vi "St temp2.vi"(11 "Station Name":string) -> ()   [LabVIEW 2019]
uses:
  Ctrl/Conveyor Action.ctl
  <vilib>/Utility/miscctls.llb/LVPointTypeDef.ctl
  Ctrl/Auto Inspection Data Name.ctl
  Ctrl/Auto Inspection Station Name2.ctl
  LLB/Message/Ctrl/MsgDataInput.ctl
  LLB/Message/Ctrl/MsgPageSelect.ctl
  LLB/Message/Ctrl/LogType.ctl
  9b7d8055-4de2-48cf-bbcb-f861e34e7884.vi
  2931b48d-cced-43b2-9067-584d882f955d.vi
  <vilib>/JDP Science/JSONtext/Variant to JSON Text.vi
  <vilib>/JDP Science/JSONtext/JSON text to Variant.vi
  LLB/Commonly VI.lvlib
  ab69a899-d2ec-4c26-af5e-ed1cd18d461c.vi
  Function/Axis/Axis_Class/SubVI/Axis Motion/Axis_Go Home.vi
  LLB/Message/MsgShowAndLog.lvlib
panel:
  in  "Table Control":string[][](table)
  out "Station Name 3":string
  in  "Enum 2":T1
  in  "Cluster":cluster{"Enum 2":T1, "Station Name 3":string}
  in  "CurrentAction":string
  in  "Status":string
  in  "Errset":bool
  out "Message":string
  out "Ring":u16(ring)
  in  "Btn_AutoRun":bool
  in  "Boolean":bool=TRUE
  in  "Btn_Home":bool
  in  "AI":T2
  in  "Tab Control":enum32{"Page 1", "Page 2"}(tab)
  in  "Enum 28":T1
  out "Station Name 29":string
  in  "Enum 27":T1
  out "Station Name 28":string
  in  "Enum 26":T1
  out "Station Name 27":string
  in  "Enum 25":T1
  out "Station Name 26":string
  in  "Enum 24":T1
  out "Station Name 25":string
  in  "Enum 23":T1
  out "Station Name 24":string
  in  "Enum 22":T1
  out "Station Name 23":string
  in  "Enum 21":T1
  out "Station Name 22":string
  in  "Enum 20":T1
  out "Station Name 21":string
  out "Station Name 19":string
  in  "Enum 18":T1
  out "Station Name 18":string
  in  "Enum 17":T1
  out "Station Name 17":string
  in  "Enum 16":T1
  out "Station Name 16":string
  in  "Enum 15":T1
  out "Station Name 15":string
  in  "Enum 14":T1
  out "Station Name 14":string
  in  "Enum 13":T1
  out "Station Name 13":string
  in  "Enum 12":T1
  out "Station Name 12":string
  in  "Enum 11":T1
  out "Station Name 11":string
  in  "Enum 10":T1
  out "Station Name 10":string
  in  "Enum 9":T1
  out "Station Name 9":string
  in  "Enum 8":T1
  out "Station Name 8":string
  in  "Enum 7":T1
  out "Station Name 7":string
  in  "Enum 6":T1
  out "Station Name 6":string
  in  "Enum 5":T1
  out "Station Name 5":string
  in  "Enum 4":T1
  out "Station Name 4":string
  in  "Enum 3":T1
  in  "Enum 19":T1
  out "Station Name 20":string
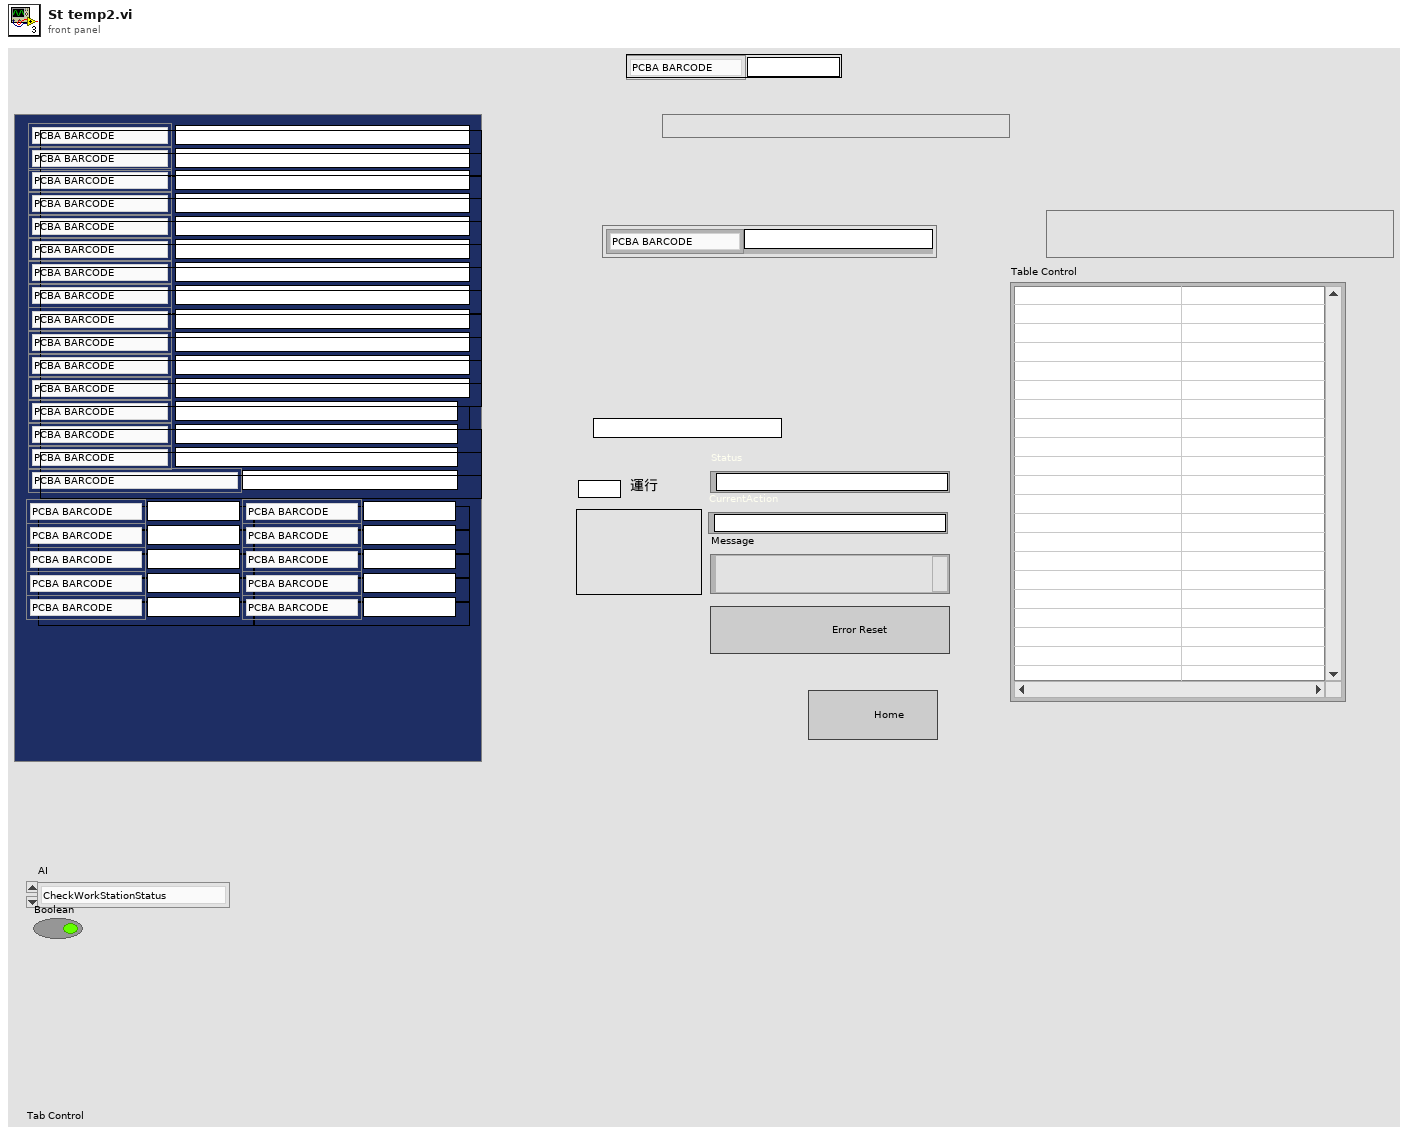
[diagram p1: front panel]
types:
  T1 = typedef "名稱資訊.ctl" = enum16{"PCBA BARCODE", "硬體(Tool初始化)", "company(Tool初始化)", "耗電流 uA(電流表)", "電池負載電壓", "晶片ID(Tool FORMAT)", "雷雕ID", "Format Status", "Programe Status", "MAC(藍芽接收器)", "ID(藍芽接收器)", "KPA(藍芽接收器)", "溫度(藍芽接收器)", "BattVol(藍芽接收器)", "RSSI(藍芽接收器)"}
  T2 = typedef "Conveyor Action.ctl" = enum16{"CheckWorkStationStatus", "Request Item In", "Check Product Ready In", "Wait Item In", "Check SlowSignal And Slow", "Check Arrive", "Rise Tray", "FixTray", "Imform Robot", "Wait Robot Imform", "DropTray Imform Out", "Wait Request ", "Flow Out"}
  T3 = enum8{"Enabled", "Disabled", "Disabled and Grayed Out"}
  T4 = typedef "LVPointTypeDef.ctl" = cluster{"Horizontal":i16, "Vertical":i16}
  T5 = typedef "MsgDataInput.ctl" = cluster{"MsgPageSelect":T6, "LogType":T7, "Msg":string, "Time":string}
  T6 = typedef "MsgShowAndLog.lvlib/MsgPageSelect.ctl" = enum16{"System", "Comm", "IO", "Action", "Alarm"}
  T7 = typedef "MsgShowAndLog.lvlib/LogType.ctl" = enum16{"Auto", "Manual", "Handshake", "Error"}
  T8 = typedef "Auto Inspection Station Name2.ctl" = enum16{"S1Barcode", "S2Measure", "S3Measure", "S4Measure", "S5Measure", "S11_LaserCheck"}
  T9 = typedef "Auto Inspection Data Name.ctl" = enum16{"LocalRun", "ItemSN(TimeCode)", "CurrentAction", "Error", "Data", "OKNG", "電壓值", "電壓值判斷", "電流值", "電流值判斷", "Laser Data", "Laser OK", "Laser NG", "StationNO"}
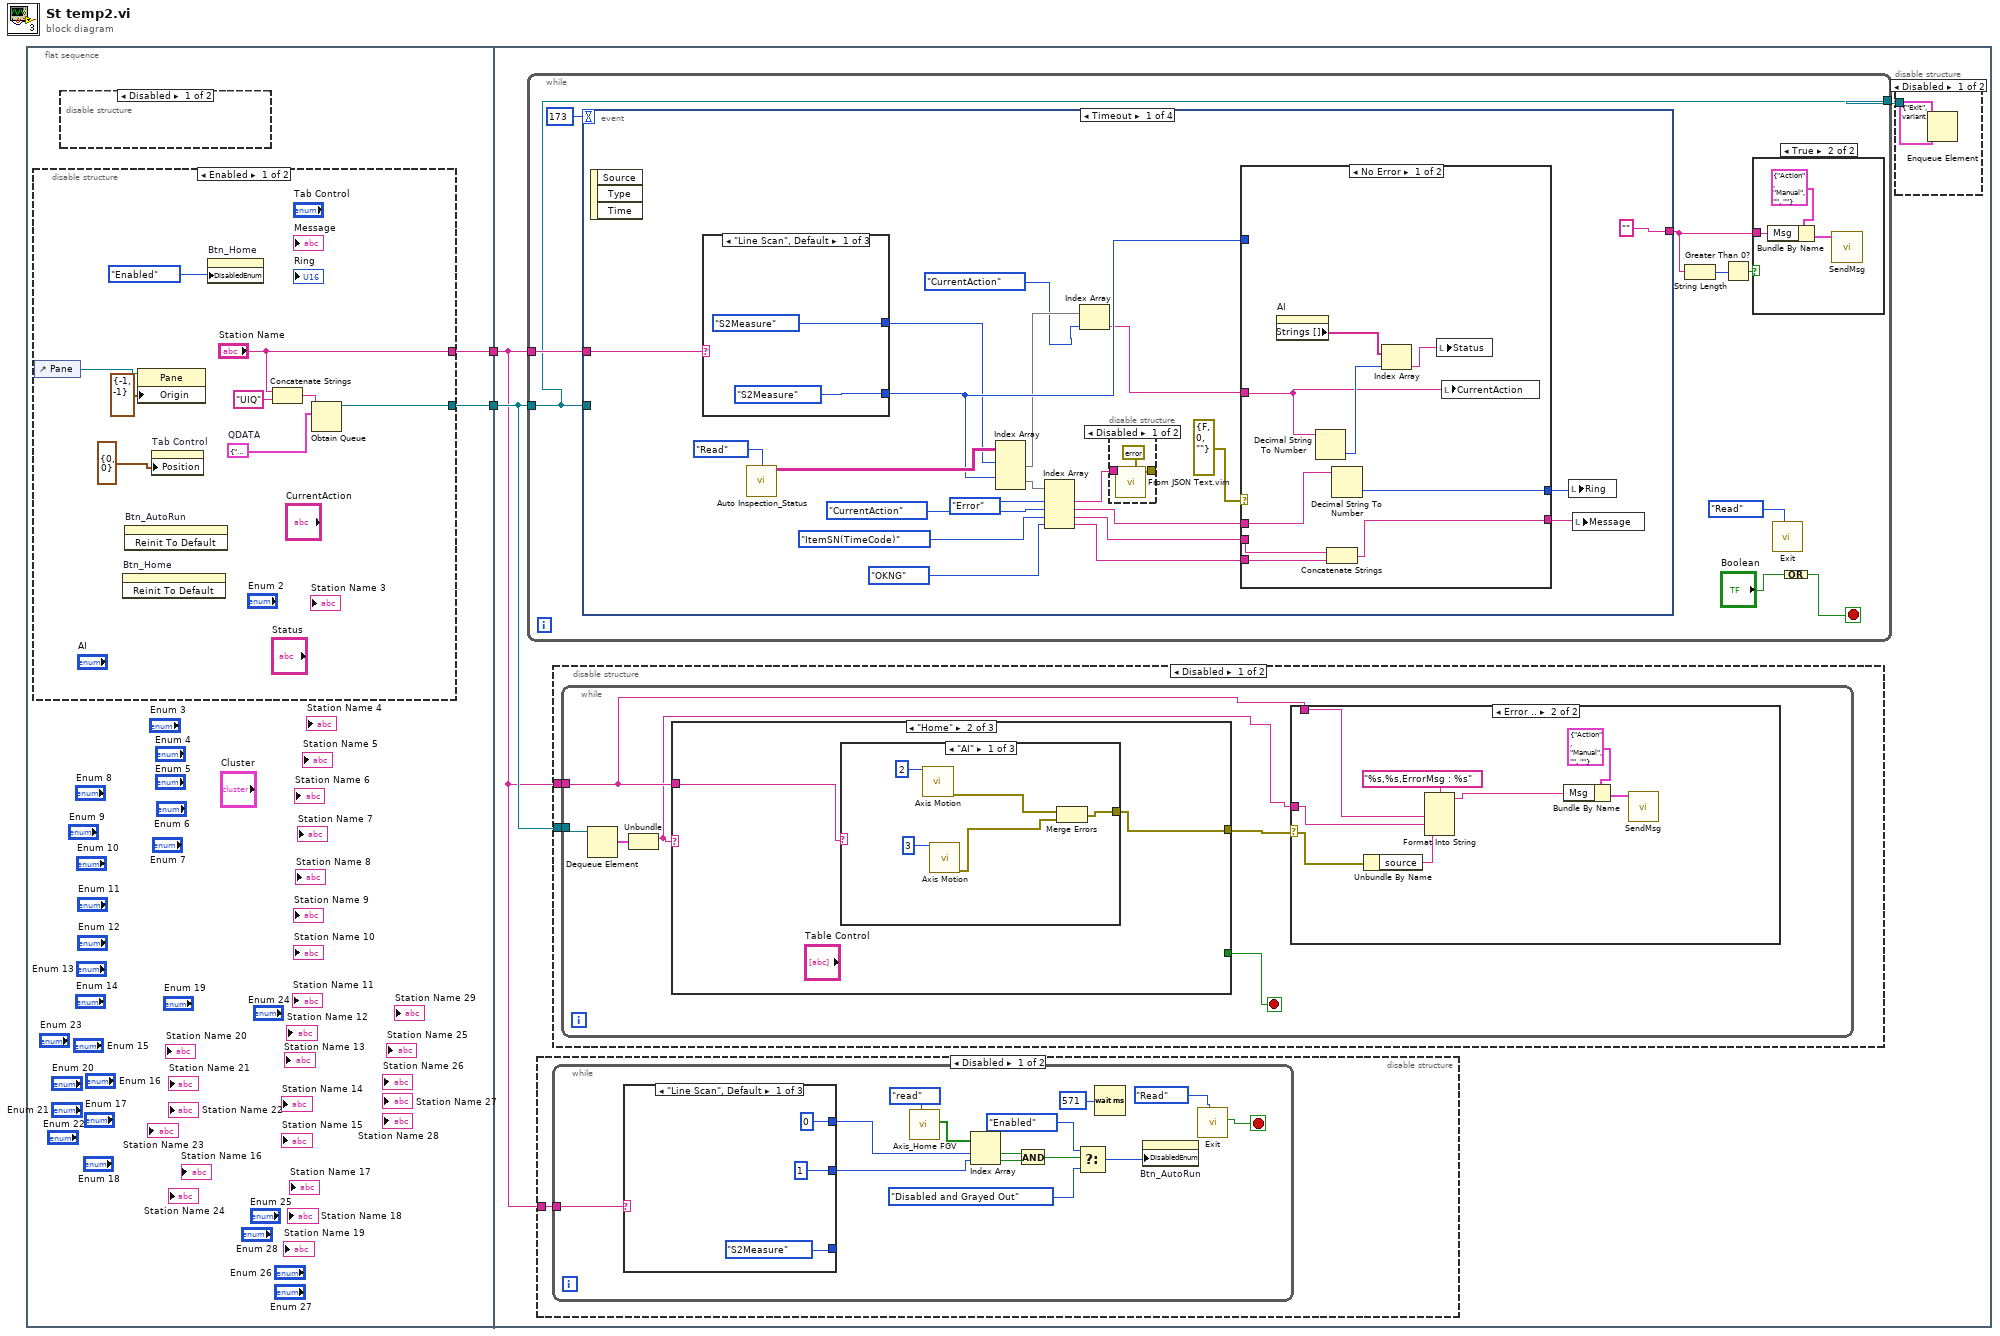
[diagram p0: block diagram]
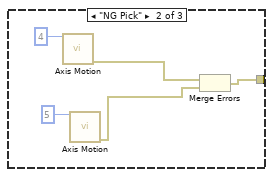
[diagram p7: hidden frame]
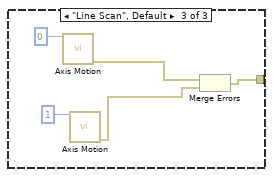
[diagram p8: hidden frame]
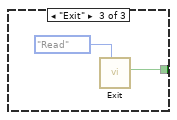
[diagram p9: hidden frame]
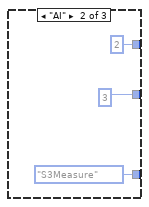
[diagram p11: hidden frame]
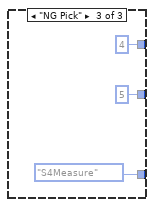
[diagram p12: hidden frame]
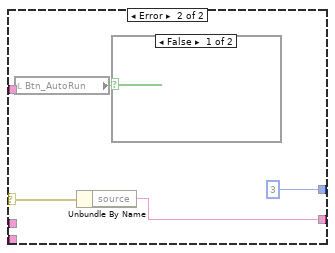
[diagram p16: hidden frame]
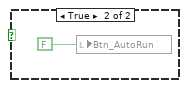
[diagram p17: hidden frame]
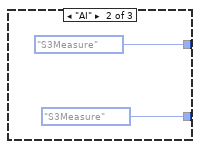
[diagram p18: hidden frame]
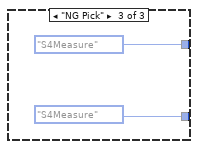
[diagram p19: hidden frame]
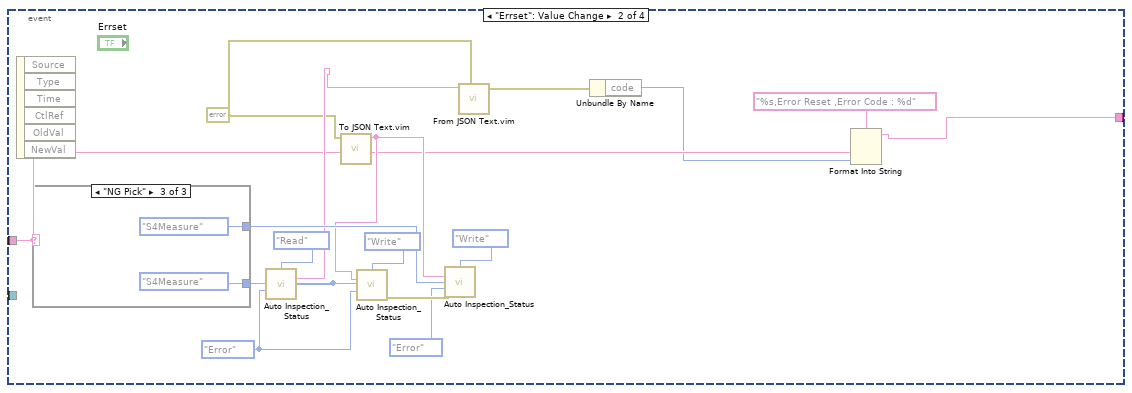
[diagram p20: hidden frame]
diagram:
  n1 = flat-sequence {
    tunnel: [w4] -> w2
    tunnel: [w3] -> w1
    tunnel: w2 -> [w14]
    tunnel: w1 -> [w16]
    frame #0 {
      n2 = disable-structure shown="Enabled" {
        disable-tunnel: ["Station Name" _] -> w4
        disable-tunnel: [w5 _] -> w3
        frame Enabled {
          w6 = cluster{"ACT":string, "DATA":variant} {"ACT"="", "DATA"=variant}  # QDATA
          n3 = control-ref of="Pane"() -> (w13:refnum<vi>)
          n4 = invoke on="Btn_Home" class="Bool" method="Reinit To Default"() -> ()  [unwired: 3 in, 3 out]
          n5 = invoke on="Btn_AutoRun" class="Bool (strict)" method="Reinit To Default"() -> ()  [unwired: 3 in, 3 out]
          n6 = property class="Pane"(reference=w13, "Origin"=T4 {"Horizontal"=-1, "Vertical"=-1}) -> ()  [unwired: 1 in, 2 out]
          n7 = property on="Tab Control" class="TabCtl (strict)"("Position"=T4 {"Horizontal"=0, "Vertical"=0} ("Origin")) -> ()  [unwired: 2 in, 2 out]
          n8 = property on="Btn_Home" class="Bool"("DisabledEnum"=T3."Enabled" ("Disabled")) -> ()  [unwired: 2 in, 2 out]
          n9 = Concatenate Strings("Station Name", "UIQ" ("string")) -> (w7:string)
          n10 = Obtain Queue(name (unnamed)=w7, element data type=w6) -> (queue out=w5:refnum<queue>)  [unwired: 3 in, 2 out]
        }
        frame Disabled {
        }
      }
      n11 = disable-structure shown="Disabled" {
        frame Disabled {
        }
        frame Enabled {
        }
      }
    }
    frame #1 {
      n12 = while {
        tunnel: w14 -> [w84]
        tunnel: w16 -> [w83]
        tunnel: [w83] -> w15
        stop <- w78 stop-if-true
        n13 = event shown="[0] Timeout" {
          selector: _ -> [_ _ _ _]
          dyn-events: _ -> [_ _ _ _]
          timeout: 173 -> [_ _ _ _]
          tunnel: w84 -> [w110 w136 w157 w184]
          tunnel: w83 -> [_ _ _ w183]
          tunnel: ["" w134 w159 w186] -> w82
          event Timeout {
            n14 = event-data() -> ()  [unwired: 1 in, 3 out]
            n15 = case shown="\"Line Scan\", Default" w110 {
              tunnel: [Auto_Inspection_Station_Name2."S2Measure" ("Station") Auto_Inspection_Station_Name2."S3Measure" ("Station") Auto_Inspection_Station_Name2."S4Measure" ("Station")] -> w98
              tunnel: [Auto_Inspection_Station_Name2."S2Measure" ("Station") Auto_Inspection_Station_Name2."S3Measure" ("Station") Auto_Inspection_Station_Name2."S4Measure" ("Station")] -> w97
              frame "Line Scan", Default {
              }
              frame "AI" {
              }
              frame "NG Pick" {
              }
            }
            n16 = call "Auto Inspection_Status.vi"("Action"=enum16{"Initial", "Write", "Read"}."Read") -> ("Table Control"=w109:string[][])  [unwired: 12 in, 2 out]
            n17 = Index Array(array=w109, index (row) #1=w97, index (row) #2=w98) -> (element #1=w96:string[], element #2=w108:string[])  [unwired: 2 in]
            n18 = Index Array(array=w108, index #1=Auto_Inspection_Data_Name."Error" ("Data"), index #2=Auto_Inspection_Data_Name."CurrentAction" ("Data"), index #3=Auto_Inspection_Data_Name."ItemSN(TimeCode)" ("Data"), index #4=Auto_Inspection_Data_Name."OKNG" ("Data")) -> (element #1=w105:string, element #2=w104:string, element #3=w100:string, element #4=w92:string)
            n19 = Index Array(array=w96, index=Auto_Inspection_Data_Name."CurrentAction" ("Data")) -> (element=w94:string)
            n20 = disable-structure shown="Disabled" {
              disable-tunnel: w105 -> [w113 _]
              disable-tunnel: [w112 _] -> _
              frame Disabled {
                n21 = call "From JSON Text.vim"("Data Type and Default Value"=errorcluster {"status"=FALSE, "code"=0, "source"=""} ("error constant"), "JSON"=w113) -> ("Data out"=w112:errorcluster)  [unwired: 8 in, 1 out]
              }
              frame Enabled {
              }
            }
            n22 = case shown="No Error" errorcluster {"status"=FALSE, "code"=0, "source"=""} ("error IO") {
              selector: errorcluster {"status"=FALSE, "code"=0, "source"=""} ("error IO") -> [_ w125]
              tunnel: w104 -> [w122 _]
              tunnel: [w121 3] -> w103
              tunnel: [w115 w124] -> w101
              tunnel: w100 -> [w116 _]
              tunnel: w98 -> [_ _]
              tunnel: w94 -> [w117 _]
              tunnel: w92 -> [w114 _]
              frame No Error {
                n23 = property on="AI" class="Enum (strict)"() -> ("Strings []"=w120:string[])  [unwired: 2 in, 2 out]
                n24 = Decimal String To Number(string=w117) -> (number=w119:i32)  [unwired: 2 in, 1 out]
                n25 = Concatenate Strings(w116, w114) -> (w115:string)
                n26 = Decimal String To Number(string=w122) -> (number=w121:i32)  [unwired: 2 in, 1 out]
                n27 = Index Array(array=w120, index=w119) -> (element=w118:string)
                n28 = local write "Status"(w118) -> ()
                n29 = local write "CurrentAction"(w117) -> ()
              }
              frame Error {
                n30 = local read "Btn_AutoRun"() -> (w123:bool)
                n31 = Unbundle By Name(w125) -> ("source"=w124:string)
                n32 = case shown="False" w123 {
                  frame False {
                  }
                  frame True {
                    n33 = local write "Btn_AutoRun"(FALSE) -> ()
                  }
                }
              }
            }
            n34 = local write "Ring"(w103) -> ()
            n35 = local write "Message"(w101) -> ()
          }
          event "Errset": Value Change {
            w138 = errorcluster {"status"=FALSE, "code"=0, "source"=""} ("error constant")
            w140 = Auto_Inspection_Data_Name."Error" ("Data")
            n36 = event-data() -> ()  [unwired: 1 in, 6 out]
            n37 = case shown="\"NG Pick\"" w136 {
              tunnel: [Auto_Inspection_Station_Name2."S2Measure" ("Station") Auto_Inspection_Station_Name2."S3Measure" ("Station") Auto_Inspection_Station_Name2."S4Measure" ("Station")] -> w141
              tunnel: [Auto_Inspection_Station_Name2."S2Measure" ("Station") Auto_Inspection_Station_Name2."S3Measure" ("Station") Auto_Inspection_Station_Name2."S4Measure" ("Station")] -> w146
              frame "Line Scan", Default {
              }
              frame "AI" {
              }
              frame "NG Pick" {
              }
            }
            n38 = call "Auto Inspection_Status.vi"("Action"=enum16{"Initial", "Write", "Read"}."Read", "Station"=w141, "Data"=w140) -> ("DataOut"=w139:string)  [unwired: 10 in, 2 out]
            n39 = call "To JSON Text.vim"("Anything"=w138) -> ("<JSON>"=w144:string)  [unwired: 9 in, 1 out]
            n40 = call "Auto Inspection_Status.vi"("Action"=enum16{"Initial", "Write", "Read"}."Write", "DataIn"=w144, "Station"=w141, "Data"=w140) -> ("error out"=w147:errorcluster)  [unwired: 9 in, 2 out]
            n41 = call "Auto Inspection_Status.vi"("Action"=enum16{"Initial", "Write", "Read"}."Write", "DataIn"=w144, "Station"=w146, "Data"=Auto_Inspection_Data_Name."Error", "error in"=w147) -> ()  [unwired: 8 in, 3 out]
            n42 = call "From JSON Text.vim"("Data Type and Default Value"=w138, "JSON"=w139) -> ("Data out"=w137:errorcluster)  [unwired: 8 in, 1 out]
            n43 = Unbundle By Name(w137) -> ("code"=w135:i32)
            n44 = Format Into String(format string="%s,Error Reset ,Error Code : %d", w136, w135) -> (resulting string=w134:string)  [unwired: 2 in, 1 out]
          }
          event "Btn_AutoRun": Value Change {
            w163 = Auto_Inspection_Data_Name."LocalRun" ("Data")
            n45 = event-data() -> ("NewVal"=w156:bool)  [unwired: 1 in, 5 out]
            n46 = case shown="\"NG Pick\"" w157 {
              tunnel: [Auto_Inspection_Station_Name2."S2Measure" ("Station") Auto_Inspection_Station_Name2."S3Measure" ("Station") Auto_Inspection_Station_Name2."S4Measure" ("Station")] -> w164
              tunnel: [Auto_Inspection_Station_Name2."S2Measure" ("Station") Auto_Inspection_Station_Name2."S3Measure" ("Station") Auto_Inspection_Station_Name2."S4Measure" ("Station")] -> w160
              frame "Line Scan", Default {
              }
              frame "AI" {
              }
              frame "NG Pick" {
              }
            }
            n47 = Select(t="1", s=w156, f="0") -> (s? t:f=w161:string)
            n48 = Select(t=T3."Disabled and Grayed Out" ("Disabled"), s=w156, f=T3."Enabled" ("Disabled")) -> (s? t:f=w168:T3)
            n49 = property on="Btn_Home" class="Bool"("DisabledEnum"=w168) -> ()  [unwired: 2 in, 2 out]
            n50 = call "Auto Inspection_Status.vi"("Action"=enum16{"Initial", "Write", "Read"}."Write", "DataIn"=w161, "Station"=w164, "Data"=w163) -> ("error out"=w162:errorcluster)  [unwired: 9 in, 2 out]
            n51 = disable-structure shown="Enabled" {
              disable-tunnel: w163 -> [w174 _]
              disable-tunnel: w162 -> [w173 _]
              disable-tunnel: w161 -> [w172 _]
              disable-tunnel: w160 -> [w171 _]
              frame Disabled {
                n52 = call "Auto Inspection_Status.vi"("Action"=enum16{"Initial", "Write", "Read"}."Write", "DataIn"=w172, "Station"=w171, "Data"=w174, "error in"=w173) -> ()  [unwired: 8 in, 3 out]
              }
              frame Enabled {
              }
            }
            n53 = Format Into String(format string="%s,Auto Run,%s", w157, w156) -> (resulting string=w159:string)  [unwired: 2 in, 1 out]
          }
          event "Btn_Home": Value Change {
            n54 = event-data() -> ()  [unwired: 1 in, 6 out]
            n55 = Enqueue Element(queue=w183, element=cluster{"ACT":string, "DATA":variant} {"ACT"="Home", "DATA"=variant}) -> ()  [unwired: 2 in, 3 out]
            n56 = Format Into String(format string="%s,Search HM", w184) -> (resulting string=w186:string)  [unwired: 2 in, 1 out]
          }
        }
        n57 = String Length(string=w82) -> (length=w81:i32)
        n58 = Greater Than 0?(x=w81) -> (x > 0?=w80:bool)
        n59 = case shown="True" w80 {
          tunnel: w82 -> [_ w87]
          frame False {
          }
          frame True {
            n60 = Bundle By Name(cluster=T5 {"MsgPageSelect"=enum."Action", "LogType"=enum."Manual", "Msg"="", "Time"=""} ("DataIn"), "Msg"=w87) -> (w88:T5)
            n61 = call "SendMsg.vi"("DataIn"=w88) -> ()  [unwired: 10 in, 1 out]
          }
        }
        n62 = call "Exit.vi"("Enum"=enum16{"Initial", "Read", "Write"}."Read") -> ()  [unwired: 10 in, 1 out]
        n63 = Compound Arithmetic op=OR("Boolean") -> (w78:bool)
      }
      n64 = disable-structure shown="Disabled" {
        disable-tunnel: w14 -> [w54 _]
        frame Disabled {
          n65 = while {
            tunnel: w54 -> [w66]
            stop <- w68 stop-if-true
            n66 = case shown="\"Line Scan\", Default" w66 {
              tunnel: [Auto_Inspection_Station_Name2."S2Measure" ("Station") Auto_Inspection_Station_Name2."S3Measure" ("Station") Auto_Inspection_Station_Name2."S4Measure" ("Station")] -> _
              tunnel: [0 2 4] -> w63
              tunnel: [1 ("Axis") 3 5 ("Axis")] -> w62
              frame "Line Scan", Default {
              }
              frame "AI" {
              }
              frame "NG Pick" {
              }
            }
            n67 = call "Axis_Home FGV.vi"("Enum"=enum16{"Initial", "write", "read"}."read") -> ("HMSStatus"=w64:bool[])  [unwired: 9 in, 1 out]
            n68 = Index Array(array=w64, index #1=w63, index #2=w62) -> (element #1=w60:bool, element #2=w61:bool)
            n69 = And(x=w60, y=w61) -> (x .and. y?=w59:bool)
            n70 = Select(t=T3."Enabled" ("Disabled"), s=w59, f=T3."Disabled and Grayed Out" ("Disabled")) -> (s? t:f=w55:T3)
            n71 = Wait (ms)(milliseconds to wait=u32 571) -> ()  [unwired: 1 out]
            n72 = property on="Btn_AutoRun" class="Bool (strict)"("DisabledEnum"=w55) -> ()  [unwired: 2 in, 2 out]
            n73 = call "Exit.vi"("Enum"=enum16{"Initial", "Read", "Write"}."Read") -> ("ExitOut"=w68:bool)  [unwired: 10 in]
          }
        }
        frame Enabled {
        }
      }
      n74 = disable-structure shown="Disabled" {
        disable-tunnel: w16 -> [w20 _]
        disable-tunnel: w14 -> [w19 _]
        frame Disabled {
          n75 = while {
            tunnel: w20 -> [w26]
            tunnel: w19 -> [w24]
            stop <- w25 stop-if-true
            n76 = Dequeue Element(queue=w26) -> (element=w23:cluster{"ACT":string, "DATA":variant})  [unwired: 2 in, 3 out]
            n77 = Unbundle(w23) -> ("ACT"=w21:string)  [unwired: 1 out]
            n78 = case shown="\"Home\"" w21 {
              tunnel: [_ _ w52] -> w25
              tunnel: w24 -> [_ w36 _]
              tunnel: [_ w35 _] -> w22
              frame "False", Default {
              }
              frame "Home" {
                n79 = case shown="\"AI\"" w36 {
                  tunnel: [w37 w42 w47] -> w35
                  frame "AI" {
                    n80 = call-poly "Axis Motion.vi"("Axis Index"=2) -> ("error"=w39:errorcluster)  [unwired: 10 in]
                    n81 = call-poly "Axis Motion.vi"("Axis Index"=3) -> ("error"=w38:errorcluster)  [unwired: 10 in]
                    n82 = Merge Errors(w39, w38) -> (w37:errorcluster)
                  }
                  frame "NG Pick" {
                    n83 = call-poly "Axis Motion.vi"("Axis Index"=4) -> ("error"=w44:errorcluster)  [unwired: 10 in]
                    n84 = call-poly "Axis Motion.vi"("Axis Index"=5) -> ("error"=w43:errorcluster)  [unwired: 10 in]
                    n85 = Merge Errors(w44, w43) -> (w42:errorcluster)
                  }
                  frame "Line Scan", Default {
                    n86 = call-poly "Axis Motion.vi"("Axis Index"=0) -> ("error"=w49:errorcluster)  [unwired: 10 in]
                    n87 = call-poly "Axis Motion.vi"("Axis Index"=1) -> ("error"=w48:errorcluster)  [unwired: 10 in]
                    n88 = Merge Errors(w49, w48) -> (w47:errorcluster)
                  }
                }
              }
              frame "Exit" {
                n89 = call "Exit.vi"("Enum"=enum16{"Initial", "Read", "Write"}."Read") -> ("ExitOut"=w52:bool)  [unwired: 10 in]
              }
            }
            n90 = case shown="Error .." w22 {
              selector: w22 -> [_ w28]
              tunnel: w24 -> [_ w30]
              tunnel: w21 -> [_ w29]
              frame No Error {
              }
              frame Error {
                n91 = Unbundle By Name(w28) -> ("source"=w27:string)
                n92 = Format Into String(format string="%s,%s,ErrorMsg : %s", w30, w29, w27) -> (resulting string=w31:string)  [unwired: 2 in, 1 out]
                n93 = Bundle By Name(cluster=T5 {"MsgPageSelect"=enum."Action", "LogType"=enum."Manual", "Msg"="", "Time"=""} ("DataIn"), "Msg"=w31) -> (w34:T5)
                n94 = call "SendMsg.vi"("DataIn"=w34) -> ()  [unwired: 10 in, 1 out]
              }
            }
          }
        }
        frame Enabled {
        }
      }
      n95 = disable-structure shown="Disabled" {
        disable-tunnel: w15 -> [w18 _]
        frame Disabled {
          n96 = Enqueue Element(queue=w18, element=cluster{"ACT":string, "DATA":variant} {"ACT"="Exit", "DATA"=variant}) -> ()  [unwired: 2 in, 3 out]
        }
        frame Enabled {
        }
      }
    }
  }
